vi "Shared Variable Issues 2.vi"() -> ()   [LabVIEW 2011]
uses:
  <vilib>/lvdsc/NI_DSC.lvlib
panel:
  in  "network settings":T1={"use binding? (F)"=TRUE, "URL"="\\\\localhost\\vlinac\\css\\css:cos", "access type"=enum."Read/write", "buffer size"=50, "use buffering? (F)"=FALSE, "single writer? (F)"=FALSE}
  out "error out 2":errorcluster
  out "data out":dbl
  out "error out":errorcluster
  in  "stop":bool
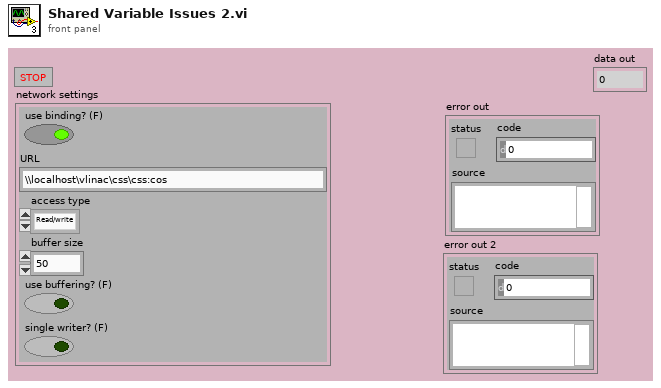
[diagram p1: front panel]
types:
  T1 = cluster{"use binding? (F)":bool, "URL":string, "access type":enum32{"Read only", "Write only", "Read/write"}, "buffer size":u32, "use buffering? (F)":bool, "single writer? (F)":bool}
  T2 = enum32{"u32BitField", "bool", "double", "string", "int8", "uint8", "int16", "uint16", "int32", "uint32", "int64", "uint64", "single", "double waveform", "int16 waveform", "array of boolean", "array of int8", "array of uint8", "array of int16", "array of uint16", "array of int32", "array of uint32", "array of int64", "array of uint64", "array of single", "array of double", "array of double waveform", "array of int16 waveform", "array of string", "variant", "timestamp", "fixed point", "custom"}
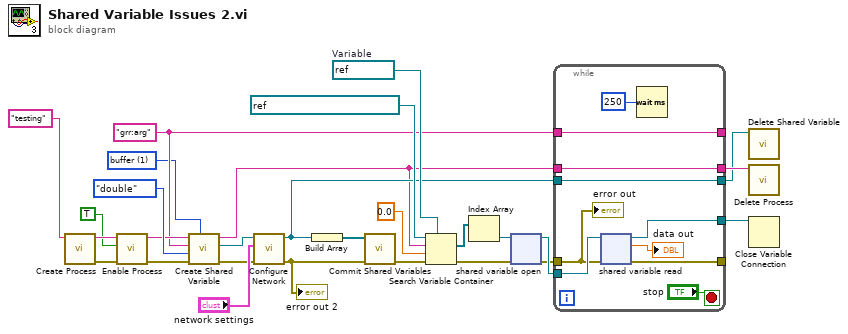
[diagram p0: block diagram]
diagram:
  w3 = u16 1 items=["commit", "buffer"] ("set mode")
  w25 = refnum<k21> refnum  # Variable
  w6 = "grr:arg" ("record name")
  n1 = call <vilib>:"Create Process.vi"("process name"="testing") -> ("error out"=w14:errorcluster, "process name out"=w17:string)  [unwired: 9 in]
  n2 = call <vilib>:"Enable Process.vi"("error in (no error)"=w14, "run?"=TRUE, "process name"=w17) -> ("error out"=w5:errorcluster, "process name out"=w16:string)  [unwired: 7 in]
  n3 = call <vilib>:"Create Shared Variable.vi"("set mode"=w3, "error in (no error)"=w5, "data type"=T2."double", "shared variable name"=w6, "process name"=w16) -> ("error out"=w4:errorcluster, "shared variable"=w11:refnum<k21>, "process name out"=w2:string)  [unwired: 4 in]
  n4 = call <vilib>:"Configure Network.vi"("error in (no error)"=w4, "network settings"="network settings", "variable reference in"=w11) -> ("error out"=w10:errorcluster, "variable reference out"=w7:refnum<k21>)  [unwired: 7 in]
  "error out 2" <- w10
  n5 = Build Array(w7) -> (w8:refnum<k21>[])
  n6 = call <vilib>:"Commit Shared Variables.vi"("error in (no error)"=w10, "shared variables"=w8) -> ("error out"=w9:errorcluster)  [unwired: 8 in, 1 out]
  n7 = Search Variable Container(7:w25, 8:w9, 9:0.0, 10:w2, 11:refnum<k21> "ni.var.psp://NDW1032/" ("container refnum in")) -> (0:w19:errorcluster, 2:w23:refnum<k21>[])  [unwired: 1 in, 1 out]
  n8 = Index Array(array=w23) -> (element=w20:refnum<k21>)  [unwired: 1 in]
  n9 = shared-variable-open(w20, w19) -> (w22:refnum<k21>, w18:errorcluster)  [unwired: 1 in]
  n10 = while {
    tunnel: w2 -> [w36]
    tunnel: [w36] -> w27
    tunnel: w7 -> [w35]
    tunnel: [w35] -> w1
    tunnel: w22 -> [w34]
    tunnel: [w32] -> w21
    tunnel: w18 -> [w30]
    tunnel: [w31] -> _
    tunnel: w6 -> [w29]
    tunnel: [w29] -> _
    stop <- "stop" stop-if-true
    n11 = shared-variable-read(w34, w30) -> (w32:refnum<k21>, w31:errorcluster, →"data out":dbl)  [unwired: 1 out]
    n12 = Wait (ms)(milliseconds to wait=u32 250) -> ()  [unwired: 1 out]
    "error out" <- w30
  }
  n13 = call <vilib>:"Delete Shared Variable.vi"("shared variable"=w1) -> ()  [unwired: 10 in, 1 out]
  n14 = call <vilib>:"Delete Process.vi"("process name"=w27) -> ()  [unwired: 10 in, 1 out]
  n15 = Close Variable Connection(11:w21) -> ()  [unwired: 1 in, 1 out]
